vi "is User Exist.vi"(8 "error in (no error)":errorcluster, 10 "username":string, 11 "[Data] Userinfo Binary in":refnum<class "[Data] Userinfo Binary.lvclass">) -> (0 "error out":errorcluster, 2 "exist?":bool, 3 "[Data] Userinfo Binary out":refnum<class "[Data] Userinfo Binary.lvclass">)   [LabVIEW 2020, in "[Data] Userinfo Binary.lvclass"]
uses:
  [Data] Userinfo Binary.lvclass
  [Data] Userinfo Binary.lvclass/[Data] Userinfo Binary.ctl
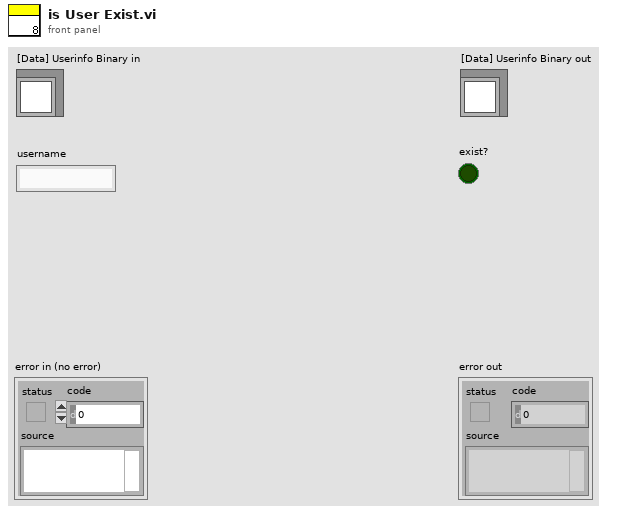
[diagram p1: front panel]
types:
  T1 = typedef "[Data] Userinfo Binary.lvclass/user info.ctl" = cluster{"password":string, "authority":i8, "department":string, "post":string, "remark":string, "create time":timestamp, "last login time":timestamp}
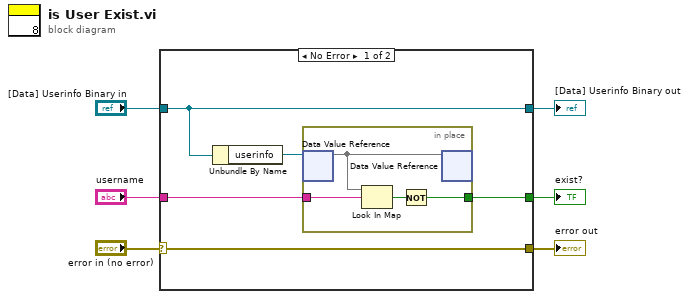
[diagram p0: block diagram]
diagram:
  n1 = case shown="No Error" "error in (no error)" {
    selector: "error in (no error)" -> [w11 w17]
    tunnel: [w11 w17] -> w5
    tunnel: [w10 w16] -> w3
    tunnel: "[Data] Userinfo Binary in" -> [w10 w16]
    tunnel: "username" -> [w9 _]
    tunnel: [w8 _] -> w1
    frame No Error {
      n2 = Unbundle By Name(w10) -> ("userinfo"=w7:refnum<data-value>)
      n3 = in-place {
        in-place-border: w9 -> [w15]
        in-place-border: [w13] -> w8
        n4 = in-place-dvr #1(w7) -> (w12:map{string, T1})  [unwired: 1 out]
        n5 = Look In Map(map=w12, key=w15) -> (key not found?=w14:bool)  [unwired: 1 in, 1 out]
        n6 = Not(x=w14) -> (.not. x?=w13:bool)
        n7 = in-place-dvr #1(w12) -> ()  [unwired: 2 out]
      }
    }
    frame Error {
    }
  }
  "error out" <- w5
  "[Data] Userinfo Binary out" <- w3
  "exist?" <- w1
